vi "IO Channels to XML.vi"() -> (0 "XML Data":string)   [LabVIEW 2013]
uses:
  Types/IO Channels.ctl
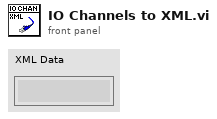
[diagram p1: front panel]
types:
  T1 = typedef "IO Channels.ctl" = cluster{"Division Input Channel":string, "Sum Input Channel":string, "X Input Channel":string, "X Output Channel":string, "Y Input Channel":string, "Y Output Channel":string, "Z Input Channel":string, "Z Output Channel":string, "Version":string}
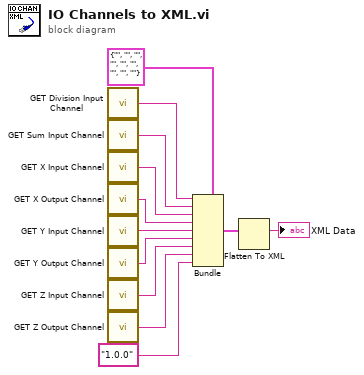
[diagram p0: block diagram]
diagram:
  n1 = call "GET Division Input Channel.vi"() -> ("Division Input Channel"=w5:string)
  n2 = call "GET Sum Input Channel.vi"() -> ("Sum Input Channel"=w6:string)
  n3 = call "GET X Input Channel.vi"() -> ("X Input Channel"=w7:string)
  n4 = call "GET X Output Channel.vi"() -> ("X Output Channel"=w8:string)
  n5 = call "GET Y Input Channel.vi"() -> ("Y Input Channel"=w10:string)
  n6 = call "GET Y Output Channel.vi"() -> ("Y Output Channel"=w9:string)
  n7 = call "GET Z Input Channel.vi"() -> ("Z Input Channel"=w3:string)
  n8 = call "GET Z Output Channel.vi"() -> ("Z Output Channel"=w2:string)
  n9 = Bundle(cluster=T1 {"Division Input Channel"="", "Sum Input Channel"="", "X Input Channel"="", "X Output Channel"="", "Y Input Channel"="", "Y Output Channel"="", "Z Input Channel"="", "Z Output Channel"="", "Version"=""} ("IO Channels"), "Division Input Channel"=w5, "Sum Input Channel"=w6, "X Input Channel"=w7, "X Output Channel"=w8, "Y Input Channel"=w10, "Y Output Channel"=w9, "Z Input Channel"=w3, "Z Output Channel"=w2, "Version"="1.0.0") -> (w12:T1)
  n10 = Flatten To XML(anything=w12) -> (xml string=→"XML Data":string)
